vi "SysInfo-Get Drives Info.vi"(11 "Error In":errorcluster) -> (8 "Array":T1[](array[typedef]), 15 "Error Out":errorcluster)   [LabVIEW 2020]
doc: "Get information about drive in specified path"
uses:
  SysInfo-Drive Info.ctl
  SysInfo-Drive Type.ctl
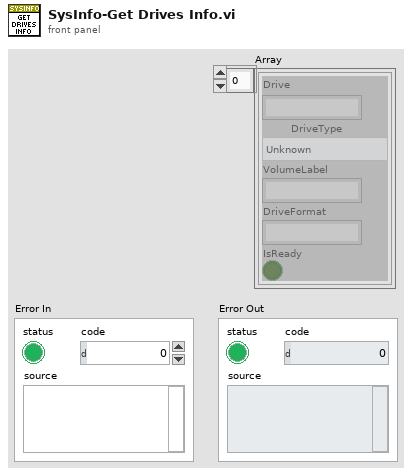
[diagram p1: front panel]
types:
  T1 = typedef "SysInfo-Drive Info.ctl" = cluster{"Drive":string, "DriveType":T2, "VolumeLabel":string, "DriveFormat":string, "IsReady":bool}
  T2 = typedef "SysInfo-Drive Type.ctl" = enum16{"Unknown", "NoRootDirectory", "Removable", "Fixed", "Network", "CDRom", "Ram"}
  T3 = cluster{"Name":string, "DriveType Ctrl":T2, "VolumeLabel":string, "DriveFormat":string, "IsReady":bool}
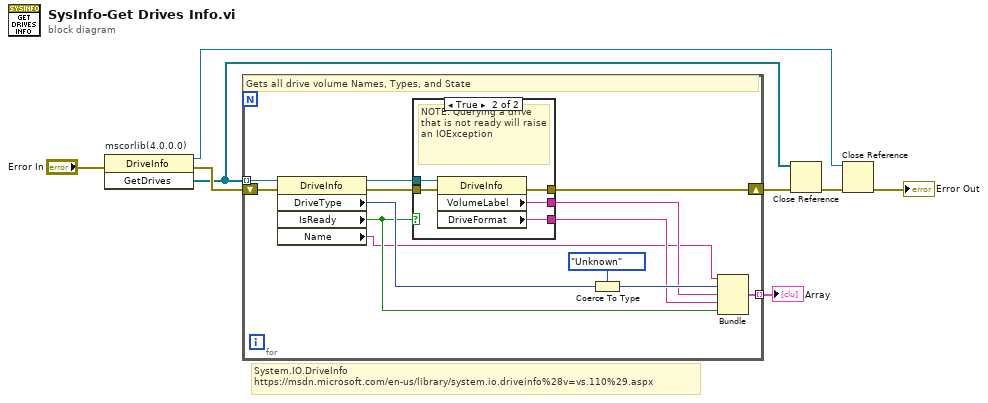
[diagram p0: block diagram]
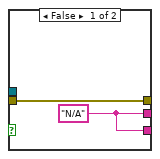
[diagram p2: hidden frame]
diagram:
  # "System.IO.DriveInfo\nhttps://msdn.microsoft.com/en-us/library/system.io.driveinfo%28v=vs.110%29.aspx"
  n1 = invoke on="mscorlib(4.0.0.0)" class="DriveInfo" method="GetDrives"(error in="Error In") -> (reference out=w4:refnum<k24>, error out=w8:errorcluster, "GetDrives"=w6:refnum<k24>[])  [unwired: 2 in]
  n2 = for {
    tunnel: w6 -> [w21] mode=indexing
    shift-right: [w16] -> w7
    shift-left: w8 -> [w20]
    tunnel: [w10] -> w1 mode=indexing
    # "Gets all drive volume Names, Types, and State"
    n3 = property class="DriveInfo"(reference=w21, error in=w20) -> (reference out=w18:refnum<k24>, error out=w17:errorcluster, "DriveType"=w19:i32, "IsReady"=w11:bool, "Name"=w9:string)
    n4 = case shown="True" w11 {
      tunnel: w18 -> [_ w28]
      tunnel: w17 -> [w23 w27]
      tunnel: [w23 w26] -> w16
      tunnel: [w22 w25] -> w13
      tunnel: [w22 w24] -> w12
      frame False {
        w22 = "N/A" ("VolumeLabel")
      }
      frame True {
        # "NOTE: Querying a drive that is not ready will raise an IOException"
        n5 = property class="DriveInfo"(reference=w28, error in=w27) -> (error out=w26:errorcluster, "VolumeLabel"=w25:string, "DriveFormat"=w24:string)  [unwired: 1 out]
      }
    }
    n6 = Coerce To Type(0:w19, 1:SysInfo-Drive_Type."Unknown" ("DriveType Ctrl")) -> (2:w14:T2)
    n7 = Bundle("Name"=w9, "DriveType Ctrl"=w14, "VolumeLabel"=w13, "DriveFormat"=w12, "IsReady"=w11) -> (w10:T3)  [unwired: 1 in]
  }
  "Array" <- w1
  n8 = Close Reference(reference=w6, error in (no error)=w7) -> (error out=w5:errorcluster)
  n9 = Close Reference(reference=w4, error in (no error)=w5) -> (error out=→"Error Out":errorcluster)
